vi "Set_ITC_Remote.vi"   [LabVIEW 2016]
uses:
  Instrument_Setup.vi
types:
  T1 = typedef "PSSetupArray.ctl" = T2[]
  T2 = typedef "PSSetup.ctl" = cluster{"Max Sweep(4.2K)":dbl[unit], "Max Sweep(2.2K)":dbl[unit], "Switch htr dly":dbl[unit], "O/P contactor?":bool, "Max Field(4.2K)":dbl[unit], "Max Field(2.2K)":dbl[unit], "Description\n":string, "Settings.vi":path, "Max lead res":dbl[unit], "IO Info":T3, "Adjust shims":bool}
  T3 = typedef "PSIO.ctl" = cluster{"Address":T4, "Version":enum16{"PS", "IPS"}}
  T4 = typedef "OxfordAddress.ctl" = cluster{"Com Port":i32, "ISOBUS Address":i32, "GPIB Address":i16, "Communication":enum16{"RS232", "ISOBUS", "GPIB", "Gateway"}}
  T5 = typedef "ILMSetup.ctl" = cluster{"Address":T4, "ILM Name":string, "Display Channel":i32[]}
  T6 = typedef "ITCIO.ctl" = cluster{"Address":T4, "Version":T7, "Ch 1 dec places":i16, "Ch 2 dec places":i16, "Ch 3 dec places":i16, "Ch1 Name":string, "Ch2 Name":string, "Ch3 Name":string}
  T7 = typedef "ITCVersion.ctl" = enum16{"ITC502", "ITC503", "ITC601"}
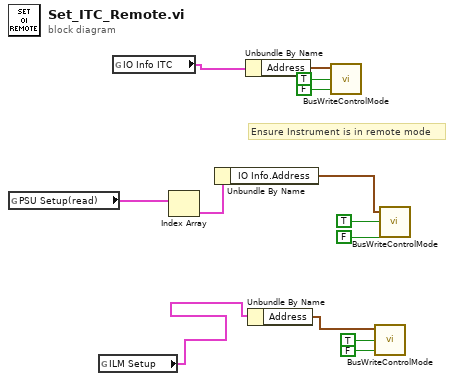
[diagram p0: block diagram]
diagram:
  # "Ensure Instrument is in remote mode"
  n1 = global read "Instrument_Setup.vi" "PSU Setup(read)"() -> (w7:T1)
  n2 = global read "Instrument_Setup.vi" "ILM Setup"() -> (w1:T5)
  n3 = global read "Instrument_Setup.vi" "IO Info ITC"() -> (w10:T6)
  n4 = Index Array(array=w7) -> (element=w6:T2)  [unwired: 1 in]
  n5 = Unbundle By Name(w6) -> ("IO Info.Address"=w5:T4)
  n6 = Unbundle By Name(w10) -> ("Address"=w13:T4)
  n7 = Unbundle By Name(w1) -> ("Address"=w2:T4)
  n8 = call "BusWriteControlMode.vi"("Locked"=FALSE, "Remote"=TRUE, "Address"=w13) -> ()  [unwired: 1 out]
  n9 = call "BusWriteControlMode.vi"("Locked"=FALSE, "Remote"=TRUE, "Address"=w2) -> ()  [unwired: 1 out]
  n10 = call "BusWriteControlMode.vi"("Locked"=FALSE, "Remote"=TRUE, "Address"=w5) -> ()  [unwired: 1 out]
